vi "Limelight.vi"() -> (0 "RightOut":dbl, 1 "LeftOut":dbl, 3 "IntakeOut":dbl)   [LabVIEW 2017]
uses:
  Robot Global Data.vi
  <vilib>/addons/control/pid/pid.llb/PID (DBL).vi
  <vilib>/addons/control/pid/NI_PID_pid.lvlib
panel:
  in  "Area Boost":dbl=30.0 format="%#_13g"
  in  "Boost":dbl=-0.5 format="%#_13g"
  in  "IntakeSpeed":dbl=-0.4 format="%#_13g"
  in  "PDistDumb":dbl=0.1 format="%#_13g"
  in  "PAngleDumb":dbl=0.04 format="%#_13g"
  in  "Distance 1":dbl=10.0 format="%#_13g"
  in  "PIDA 1":T1={"proportional gain (Kc)"=0.1, "integral time (Ti, min)"=0.0, "derivative time (Td, min)"=0.0} {"derivative time (Td, min)" format="%.3f"; "integral time (Ti, min)" format="%.3f"; "proportional gain (Kc)" format="%.3f"}
  in  "PIDX 1":T1={"proportional gain (Kc)"=0.04, "integral time (Ti, min)"=0.0, "derivative time (Td, min)"=0.0} {"derivative time (Td, min)" format="%.3f"; "integral time (Ti, min)" format="%.3f"; "proportional gain (Kc)" format="%.3f"}
  in  "MaxSpeed 1":dbl=0.4 format="%#_13g"
  in  "DriveSmart":bool
  in  "TurnSmart":bool=TRUE
  in  "Angle":dbl=10.0 format="%#_13g"
  in  "Area":dbl=80.0 format="%#_13g"
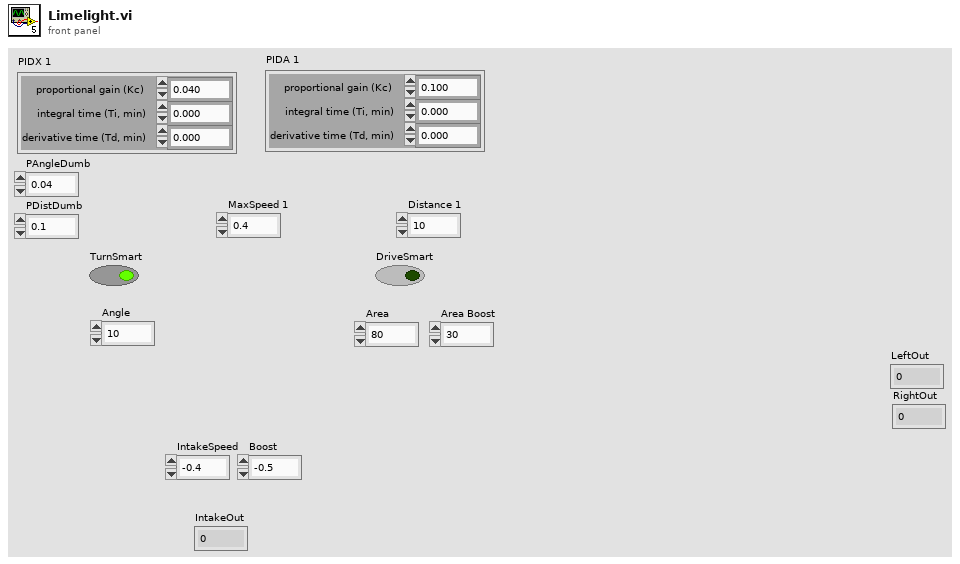
[diagram p1: front panel]
types:
  T1 = cluster{"proportional gain (Kc)":dbl, "integral time (Ti, min)":dbl, "derivative time (Td, min)":dbl}
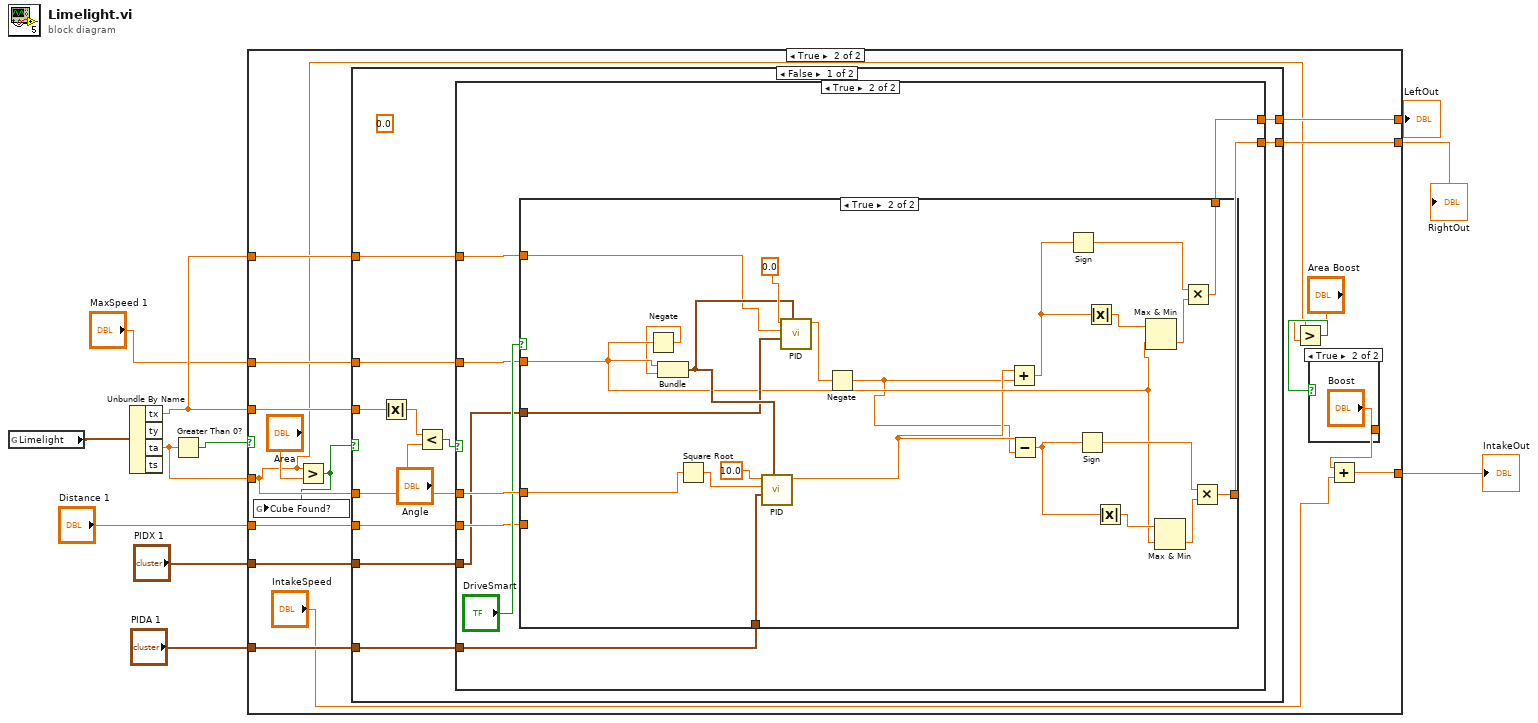
[diagram p0: block diagram]
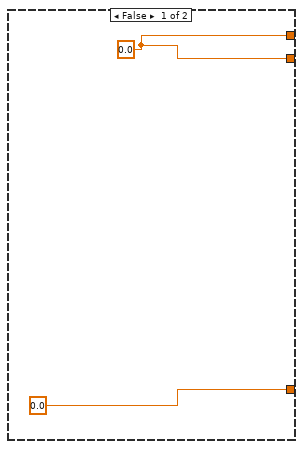
[diagram p2: hidden frame]
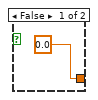
[diagram p3: hidden frame]
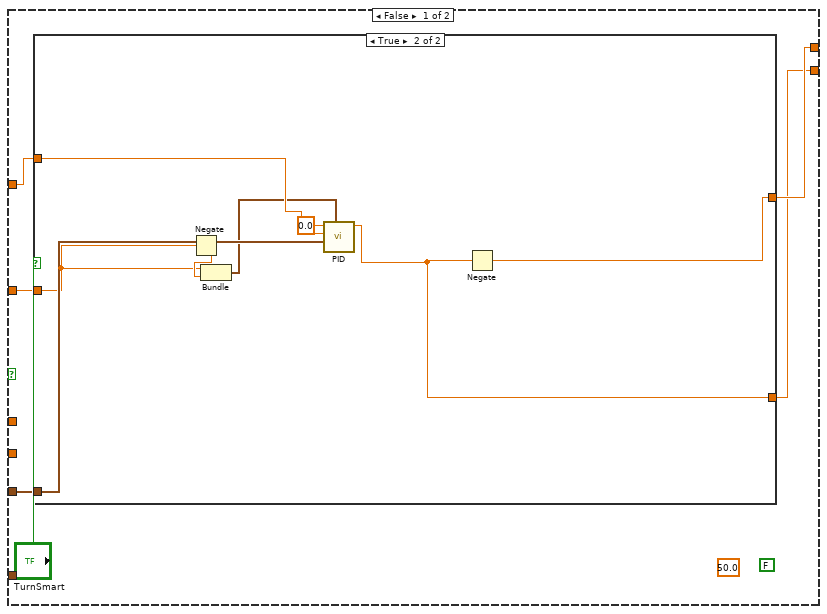
[diagram p4: hidden frame]
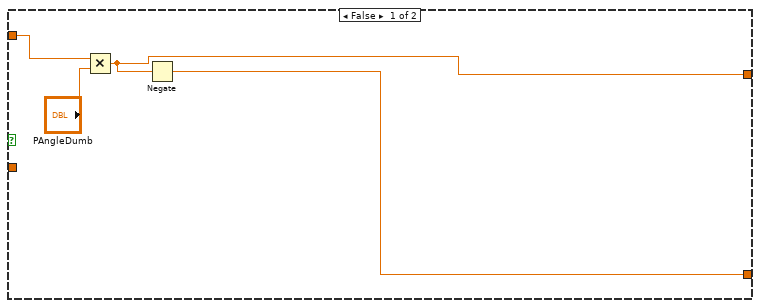
[diagram p5: hidden frame]
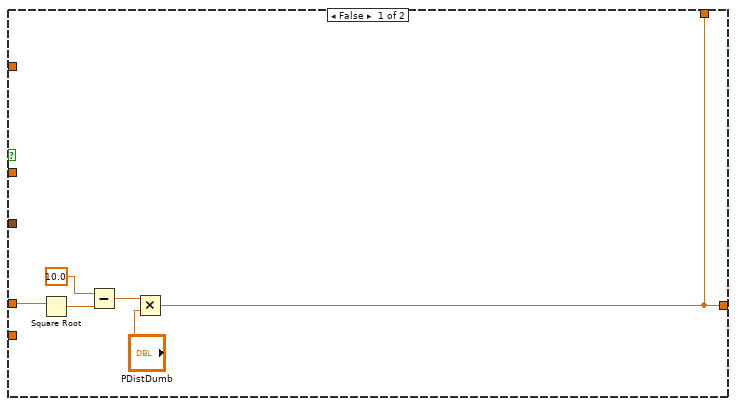
[diagram p6: hidden frame]
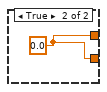
[diagram p7: hidden frame]
diagram:
  n1 = global read "Robot Global Data.vi" "Limelight"() -> (w2:cluster{"tx":dbl, "ty":dbl, "ta":dbl, "ts":dbl})
  n2 = Unbundle By Name(w2) -> ("tx"=w9:dbl, "ta"=w10:dbl)  [unwired: 2 out]
  n3 = Greater Than 0?(x=w10) -> (x > 0?=w11:bool)
  n4 = case shown="True" w11 {
    tunnel: w10 -> [_ w15]
    tunnel: w9 -> [_ w28]
    tunnel: w9 -> [_ w27]
    tunnel: [w13 w26] -> w4
    tunnel: [w13 w25] -> w3
    tunnel: "MaxSpeed 1" -> [_ w24]
    tunnel: "PIDX 1" -> [_ w23]
    tunnel: "PIDA 1" -> [_ w22]
    tunnel: "Distance 1" -> [_ w21]
    tunnel: [0.0 w20] -> w1
    frame False {
      w13 = 0.0
    }
    frame True {
      n5 = Greater?(x=w15, y="Area") -> (0:w14:bool)
      n6 = global write "Robot Global Data.vi" "Cube Found?"(w14) -> ()
      n7 = case shown="False" w14 {
        tunnel: w28 -> [w43 _]
        tunnel: w27 -> [w39 _]
        tunnel: w15 -> [w38 _]
        tunnel: [w37 w100] -> w26
        tunnel: [w36 w100] -> w25
        tunnel: w24 -> [w35 _]
        tunnel: w23 -> [w34 _]
        tunnel: w22 -> [w33 _]
        tunnel: w21 -> [w32 _]
        frame False {
          (unwired) 0.0
          n8 = Absolute Value(x=w43) -> (abs(x)=w42:dbl)
          n9 = Less?(x=w42, y="Angle") -> (x < y?=w40:bool)
          n10 = case shown="True" w40 {
            tunnel: w39 -> [w46 w70]
            tunnel: w38 -> [_ w69]
            tunnel: [w49 w68] -> w37
            tunnel: [w48 w67] -> w36
            tunnel: w35 -> [w45 w65]
            tunnel: w34 -> [w44 w62]
            tunnel: w33 -> [_ w64]
            tunnel: w32 -> [_ w63]
            frame False {
              (unwired) 50.0
              (unwired) FALSE
              n11 = case shown="True" "TurnSmart" {
                tunnel: [w51 w58] -> w49
                tunnel: [w50 w54] -> w48
                tunnel: w46 -> [w53 w60]
                tunnel: w45 -> [_ w56]
                tunnel: w44 -> [_ w59]
                frame False {
                  n12 = Multiply(x=w53, y="PAngleDumb") -> (x*y=w51:dbl)
                  n13 = Negate(x=w51) -> (-x=w50:dbl)
                }
                frame True {
                  n14 = Negate(x=w56) -> (-x=w57:dbl)
                  n15 = Bundle("MaxSpeed 1"=w56, w57) -> (w55:cluster{"MaxSpeed 1":dbl, dbl})  [unwired: 1 in]
                  n16 = call-poly <vilib>:"PID.vi"("output range"=w55, "PID gains"=w59, "process variable"=w60, "setpoint"=0.0) -> ("output"=w54:dbl)  [unwired: 6 in, 1 out]
                  n17 = Negate(x=w54) -> (-x=w58:dbl)
                }
              }
            }
            frame True {
              n18 = case shown="True" "DriveSmart" {
                tunnel: w70 -> [_ w89]
                tunnel: w69 -> [w76 w88]
                tunnel: [w72 w87] -> w68
                tunnel: [w72 w78] -> w67
                tunnel: w65 -> [_ w83]
                tunnel: w64 -> [_ w86]
                tunnel: w63 -> [_ _]
                tunnel: w62 -> [_ w85]
                frame False {
                  n19 = Square Root(x=w76) -> (sqrt(x)=w74:dbl)
                  n20 = Subtract(x=10.0, y=w74) -> (x-y=w71:dbl)
                  n21 = Multiply(x=w71, y="PDistDumb") -> (x*y=w72:dbl)
                }
                frame True {
                  n22 = Negate(x=w83) -> (-x=w82:dbl)
                  n23 = Bundle("MaxSpeed 1"=w83, w82) -> (w90:cluster{"MaxSpeed 1":dbl, dbl})  [unwired: 1 in]
                  n24 = Square Root(x=w88) -> (sqrt(x)=w80:dbl)
                  n25 = call-poly <vilib>:"PID.vi"("output range"=w90, "PID gains"=w86, "process variable"=w80, "setpoint"=10.0) -> ("output"=w81:dbl)  [unwired: 6 in, 1 out]
                  n26 = call-poly <vilib>:"PID.vi"("output range"=w90, "PID gains"=w85, "process variable"=w89, "setpoint"=0.0) -> ("output"=w84:dbl)  [unwired: 6 in, 1 out]
                  n27 = Negate(x=w84) -> (-x=w77:dbl)
                  n28 = Add(x=w81, y=w77) -> (x+y=w99:dbl)
                  n29 = Subtract(x=w81, y=w77) -> (x-y=w92:dbl)
                  n30 = Sign(1:w99) -> (0:w96:dbl)
                  n31 = Sign(1:w92) -> (0:w93:dbl)
                  n32 = Absolute Value(x=w99) -> (abs(x)=w98:dbl)
                  n33 = Absolute Value(x=w92) -> (abs(x)=w95:dbl)
                  n34 = Max & Min(x=w98, y=w83) -> (min(x,y)=w97:dbl)  [unwired: 1 out]
                  n35 = Max & Min(x=w95, y=w83) -> (min(x,y)=w94:dbl)  [unwired: 1 out]
                  n36 = Multiply(x=w96, y=w97) -> (x*y=w87:dbl)
                  n37 = Multiply(x=w93, y=w94) -> (x*y=w78:dbl)
                }
              }
            }
          }
        }
        frame True {
          w100 = 0.0
        }
      }
      n38 = Greater?(x=w15, y="Area Boost") -> (0:w17:bool)
      n39 = case shown="True" w17 {
        tunnel: [0.0 "Boost"] -> w18
        frame False {
        }
        frame True {
        }
      }
      n40 = Add(x=w18, y="IntakeSpeed") -> (x+y=w20:dbl)
    }
  }
  "LeftOut" <- w4
  "RightOut" <- w3
  "IntakeOut" <- w1
